vi "Joystick Data.vi"(0 "Joystick codrive in":dbl[](array[numeric]), 1 "Joystick Button in":bool[](array[boolean]), 2 "Xbox One In":bool[](array[boolean]), 3 "Right Joystick In":dbl, 4 "Right Buttons In":bool[](array[boolean]), 5 "Xbox One Joy In":dbl[](array[numeric]), 7 "Xbox 360 in":bool[](array[boolean]), 9 "Xbox 360 Joy In":dbl[](array[numeric]), 10 "Read/Write":T1) -> (11 "Xbox 360 Joy Out":dbl[](array[numeric]), 13 "Xbox 360 Out":bool[](array[boolean]), 14 "Joystick codrive out":dbl[](array[numeric]), 15 "Joystick Button out":bool[](array[boolean]), 16 "Xbox One Out":bool[](array[boolean]), 17 "Right Joystick Out":dbl, 18 "Right Buttons Out":bool[](array[boolean]), 19 "Xbox One Joy Out":dbl[](array[numeric]))   [LabVIEW 2018]
uses:
  Type Defs/Read Write.ctl
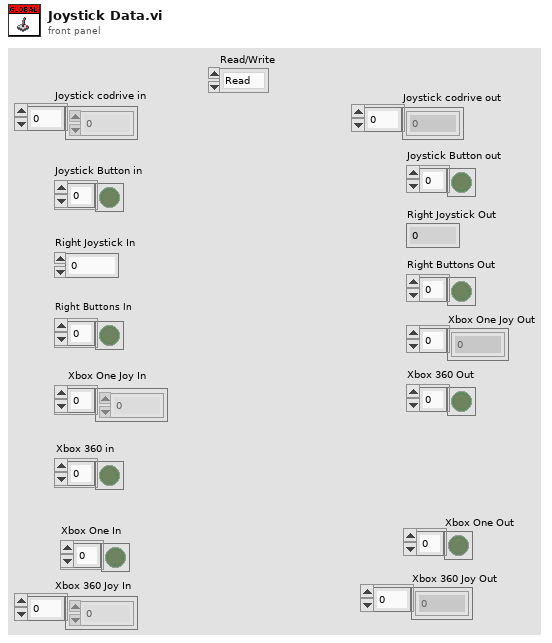
[diagram p1: front panel]
types:
  T1 = typedef "Read Write.ctl" = enum16{"Read", "Write"}
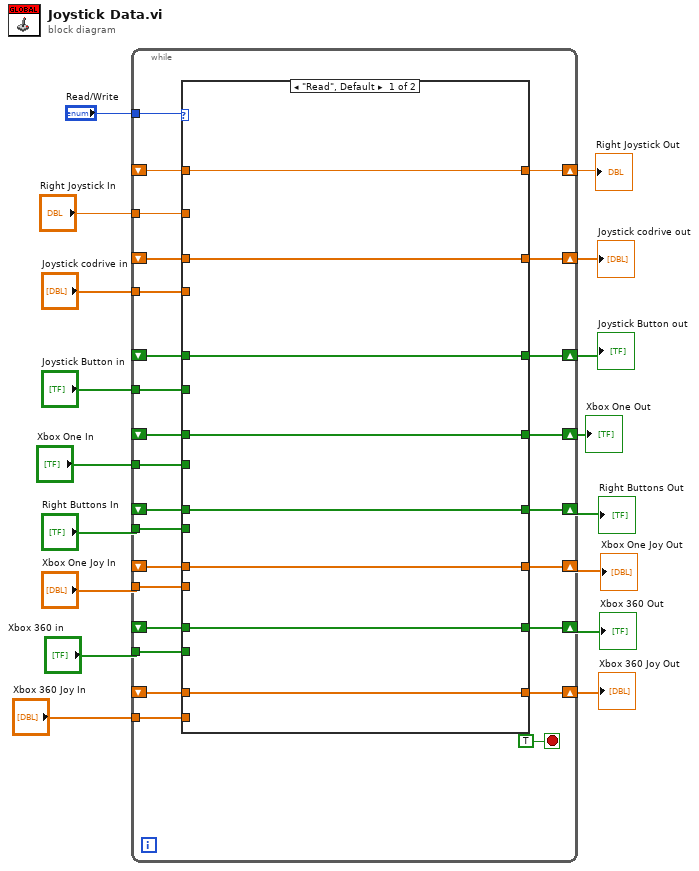
[diagram p0: block diagram]
diagram:
  n1 = while {
    shift-right: [w37] -> w12
    shift-left: _ -> [w36]
    tunnel: "Read/Write" -> [w42]
    tunnel: "Right Joystick In" -> [w41]
    tunnel: "Joystick codrive in" -> [w40]
    shift-right: [w39] -> w11
    shift-left: _ -> [w38]
    shift-right: [w34] -> w10
    shift-left: _ -> [w33]
    tunnel: "Joystick Button in" -> [w35]
    tunnel: "Right Buttons In" -> [w32]
    shift-right: [w31] -> w9
    shift-left: _ -> [w30]
    shift-right: [w28] -> w5
    shift-left: _ -> [w27]
    tunnel: "Xbox One Joy In" -> [w29]
    tunnel: "Xbox 360 in" -> [w24]
    shift-right: [w25] -> w6
    shift-left: _ -> [w26]
    tunnel: "Xbox One In" -> [w23]
    shift-right: [w22] -> w3
    shift-left: _ -> [w21]
    shift-right: [w19] -> w2
    shift-left: _ -> [w20]
    tunnel: "Xbox 360 Joy In" -> [w18]
    stop <- TRUE stop-if-true
    n2 = case shown="\"Read\", Default" w42 {
      tunnel: w41 -> [_ w59]
      tunnel: w40 -> [_ w58]
      tunnel: [w51 w58] -> w39
      tunnel: w38 -> [w51 _]
      tunnel: [w50 w59] -> w37
      tunnel: w36 -> [w50 _]
      tunnel: w35 -> [_ w57]
      tunnel: [w49 w57] -> w34
      tunnel: w33 -> [w49 _]
      tunnel: w32 -> [_ w56]
      tunnel: [w48 w56] -> w31
      tunnel: w30 -> [w48 _]
      tunnel: w29 -> [_ w55]
      tunnel: [w47 w55] -> w28
      tunnel: w27 -> [w47 _]
      tunnel: w26 -> [w46 _]
      tunnel: [w46 w54] -> w25
      tunnel: w24 -> [_ w54]
      tunnel: w23 -> [_ w53]
      tunnel: [w45 w53] -> w22
      tunnel: w21 -> [w45 _]
      tunnel: w20 -> [w44 _]
      tunnel: [w44 w52] -> w19
      tunnel: w18 -> [_ w52]
      frame "Read", Default {
      }
      frame "Write" {
      }
    }
  }
  "Right Joystick Out" <- w12
  "Joystick codrive out" <- w11
  "Joystick Button out" <- w10
  "Right Buttons Out" <- w9
  "Xbox 360 Out" <- w6
  "Xbox One Joy Out" <- w5
  "Xbox One Out" <- w3
  "Xbox 360 Joy Out" <- w2
